vi "ALP_Sub_Pattern_.vi"(5 "Last Frame":i32, 7 "First Frame":i32, 8 "error in (no error)":errorcluster, 9 "Repetitions":i32, 10 "SequenceId in":u32, 11 "DeviceIdPtr in":u32) -> (0 "error out":errorcluster, 2 "SequenceId out":u32, 3 "DeviceId":u32)   [LabVIEW 2020]
uses:
  <userlib>/alp4395/alp4395.dll
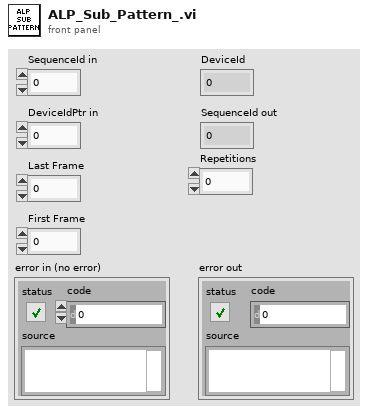
[diagram p1: front panel]
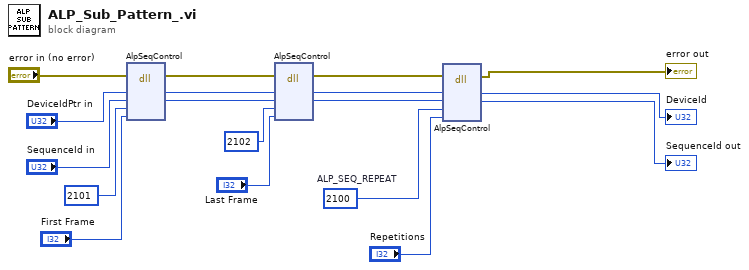
[diagram p0: block diagram]
diagram:
  w5 = 2100  # ALP_SEQ_REPEAT
  n1 = dll-call lib="C:/Program Files (x86)/National Instruments/LabVIEW 2020/user.lib/alp4395/alp4395.dll" fn="AlpSeqControl"(error in="error in (no error)", "DeviceId"="DeviceIdPtr in", "SequenceId"="SequenceId in", "ALP_FIRSTFRAME"=2101, "ControlValue"="First Frame") -> (error out=w14:errorcluster, "DeviceId"=w15:u32, "SequenceId"=w16:u32)  [unwired: 5 in, 1 out]
  n2 = dll-call lib="C:/Program Files (x86)/National Instruments/LabVIEW 2020/user.lib/alp4395/alp4395.dll" fn="AlpSeqControl"(error in=w14, "DeviceId"=w15, "SequenceId"=w16, "ALP_LASTFRAME"=2102, "ControlValue"="Last Frame") -> (error out=w8:errorcluster, "DeviceId"=w7:u32, "SequenceId"=w6:u32)  [unwired: 5 in, 1 out]
  n3 = dll-call lib="C:/Program Files (x86)/National Instruments/LabVIEW 2020/user.lib/alp4395/alp4395.dll" fn="AlpSeqControl"(error in=w8, "DeviceId"=w7, "SequenceId"=w6, "ALP_LASTFRAME"=w5, "ControlValue"="Repetitions") -> (error out=→"error out":errorcluster, "DeviceId"=→"DeviceId":u32, "SequenceId"=→"SequenceId out":u32)  [unwired: 5 in, 1 out]
